vi "Current Set.vi"(9 "Actual Number":dbl, 10 "Target":dbl, 11 "Percent ceiling":dbl=2.0) -> (2 "New Set Point":dbl)   [LabVIEW 2012]
panel:
  out "x/y":dbl
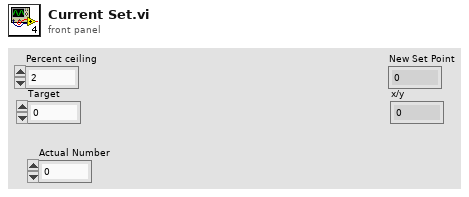
[diagram p1: front panel]
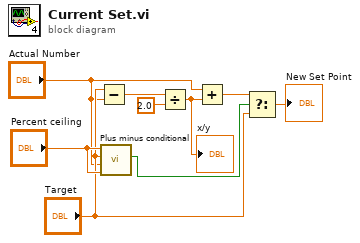
[diagram p0: block diagram]
diagram:
  n1 = Subtract(x="Target", y="Actual Number") -> (x-y=w3:dbl)
  n2 = call "Plus minus conditional.vi"("Percent Floor"="Percent ceiling", "Actual Number"="Actual Number", "Target"="Target", "Percent ceiling"="Percent ceiling") -> ("Either"=w8:bool)  [unwired: 5 in, 2 out]
  n3 = Divide(x=w3, y=2.0) -> (x/y=w1:dbl)
  "x/y" <- w1
  n4 = Add(x="Actual Number", y=w1) -> (x+y=w5:dbl)
  n5 = Select(t=w5, s=w8, f="Target") -> (s? t:f=→"New Set Point":dbl)
